vi "CS POLARIS BME DG Client.panel.vi"(8 "error in (no error)":errorcluster, 11 "object ref":refnum<vi>) -> (0 "error out":errorcluster)   [LabVIEW 2009, in "CS POLARIS BME DG Client.lvlib"]
doc: "This is the constructor of a class.\n\nLicense Agreement for this software:\n\nCopyright (C)\nGesellschaft für Schwerionenforschung, GSI\nPlanckstr. 1\n64291 Darmstadt\nGermany\n\nContact: D.Beck@gsi.de \n\nThis program is free software; you can redistribute it and/or modify it under the terms of the \nGNU General Public License as published by the Free Software Foundation; either version 2 of \nthe license, or (at your option) any later version.\n\nThis program is distributed in the hope that it will be useful, but WITHOUT ANY WARRANTY; \nwithout even the implied warranty of MERCHANTABILITY or FITNESS FOR A PARTICULAR PURPOSE. See the GNU General License for more details (http://www.gnu.org).\n\nGesellschaft für Schwerionenforschung, GSI\nPlanckstr. 1, 64291 Darmstadt, Germany\nFor all questions and ideas contact: M.Richter@gsi.de, H.Brand@gsi.de or D.Beck@gsi.de.\nLast update: 16-JUN-2004"
uses:
  CS POLARIS BME DG Client.lvlib
  CSCore/CSSystem/CoreDefs/CoreDefs.call_type.ctl
  CSCore/BaseProcess/BaseProcess.descriptor string definition.ctl
  CSCore/CSSystem/CoreDefs/CoreDefs.rawDataType.ctl
  CSCore/CSSystem/CoreLib/CoreLib.string 2 byte array.vi
  CSCore/CSSystem/CoreLib/CoreLib.byte array 2 string.vi
  CSCore/CSSystem/CoreLib/CoreLib.byte array 2 double.vi
  CSCore/CSSystem/CoreLib/CoreLib.int 2 byte array.vi
  DG Classes/BME_DG_System/ControlLevel.ctl
  CSCore/CSSystem/CSSystemLib/CSSystemLib.lvlib
  CSCore/CSSystem/CoreLib/CoreLib.lvlib
  DG Classes/BME_DG_System/BME_DG_System.lvclass
  <vilib>/gmath/NI_Gmath.lvlib
  lib.lib/UtilityLib/UtilityLib.lvlib
  CSCore/BaseProcess/BaseProcess.lvlib
panel:
  in  "deltaDelayOK":bool
  in  "call cluster in 3":T1={"Object"="", "Selector"="", "CallType"=enum."synchronous", "Async Object"="", "Async Selector"="", "Data Descriptor"="", "Data"=[], "Error #"=0, "Expire"=0}
  out "abs. Delay":dbl
  in  "call cluster in 8":T1={"Object"="", "Selector"="", "CallType"=enum."synchronous", "Async Object"="", "Async Selector"="", "Data Descriptor"="", "Data"=[], "Error #"=0, "Expire"=0}
  in  "Old Delay Formula":string
  in  "call cluster in 7":T1={"Object"="", "Selector"="", "CallType"=enum."synchronous", "Async Object"="", "Async Selector"="", "Data Descriptor"="", "Data"=[], "Error #"=0, "Expire"=0}
  in  "call cluster in 6":T1={"Object"="", "Selector"="", "CallType"=enum."synchronous", "Async Object"="", "Async Selector"="", "Data Descriptor"="", "Data"=[], "Error #"=0, "Expire"=0}
  in  "call cluster in 5":T1={"Object"="", "Selector"="", "CallType"=enum."synchronous", "Async Object"="", "Async Selector"="", "Data Descriptor"="", "Data"=[], "Error #"=0, "Expire"=0}
  in  "call cluster in 4":T1={"Object"="", "Selector"="", "CallType"=enum."synchronous", "Async Object"="", "Async Selector"="", "Data Descriptor"="", "Data"=[], "Error #"=0, "Expire"=0}
  out "Control?":bool
  in  "Tabs":enum32{"Simple", "Expert", "State"}(tab)
  out "cur. delay":dbl format="%#.9g"
  out "Ref. Chnl":string
  out "new delay":dbl format="%#.9g"
  in  "Continiously":bool
  out "Current Formula(µs)":string
  in  "ms":i32
  in  "µs":i32 min=-1000 max=1000
  in  "ns":i32 min=-1000 max=1000
  in  "Set Delay":bool
  in  "sec":i32
  in  "ps":i32 min=-1000 max=1000
  out "next common shot(s)":dbl caption="update in (s)"
  out "Out. Modulo":i32
  in  "New Modulo":i32
  in  "SetOutputMod":bool caption="Set"
  out "lockinfo":string caption="cntrl locked by"
  in  "Select ref. Chnl":u16(ring)
  out "cmd error":errorcluster
  in  "call cluster in 2":T1={"Object"="", "Selector"="", "CallType"=enum."synchronous", "Async Object"="", "Async Selector"="", "Data Descriptor"="", "Data"=[], "Error #"=0, "Expire"=0}
  in  "call cluster in":T1={"Object"="", "Selector"="", "CallType"=enum."synchronous", "Async Object"="", "Async Selector"="", "Data Descriptor"="", "Data"=[], "Error #"=0, "Expire"=0}
  out "State":i32
  out "Next Shot in (s)":dbl format="%#.1f"
  out "Rep. Rate (s)":dbl
  out "Active?":bool
  out "Channel":string
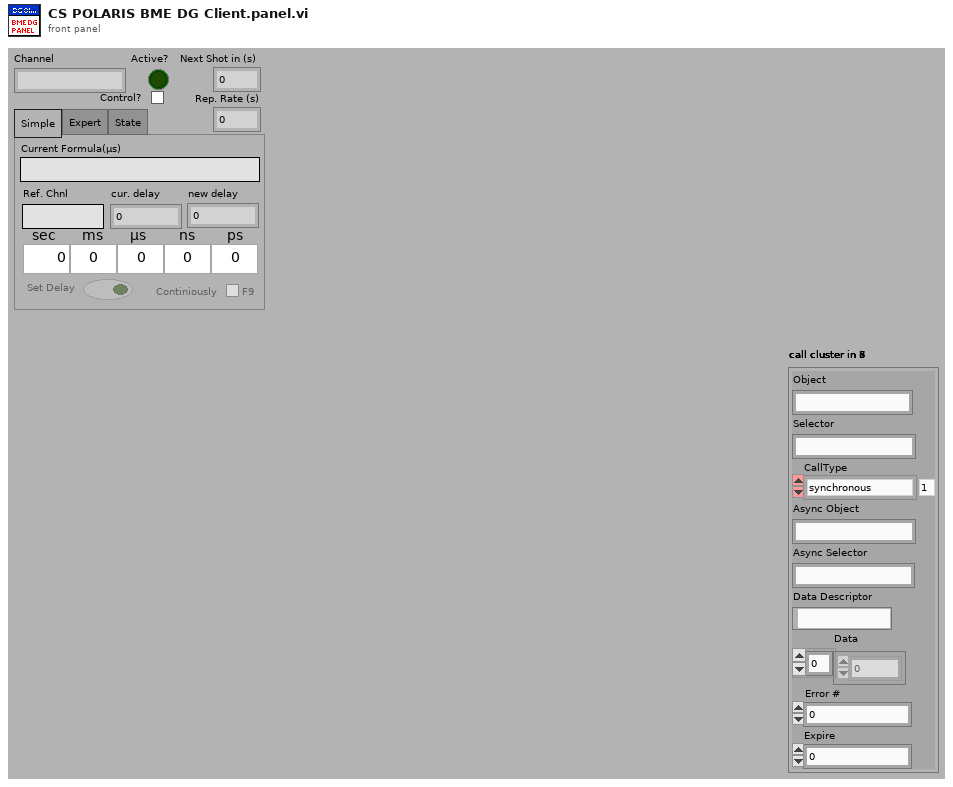
[diagram p1: front panel]
types:
  T1 = typedef "CoreDefs.call_type.ctl" = cluster{"Object":string, "Selector":string, "CallType":enum16{"simple", "synchronous", "asynchronous"}, "Async Object":string, "Async Selector":string, "Data Descriptor":T2, "Data":T3, "Error #":i32, "Expire":u32}
  T2 = typedef "BaseProcess.lvlib/BaseProcess.descriptor string definition.ctl" = string
  T3 = typedef "CoreDefs.rawDataType.ctl" = i8[]
  T4 = enum8{"Enabled", "Disabled", "Disabled and Grayed Out"}
  T5 = typedef "CS POLARIS BME DG Client.lvlib/CS POLARIS BME DG Client.i attribute.ctl" = cluster{"Delay Formula Ref":refnum<vi>, "Active Ref":refnum<vi>, "OutputModulo Ref":refnum<vi>, "Rep Rate Ref":refnum<vi>, "Next Shot Ref":refnum<vi>, "Error Ref":refnum<vi>, "Switch Ref":refnum<vi>, "New Delay Formula Ref":refnum<vi>, "New OutputModulo Ref ":refnum<vi>, "Channel":string, "CS DG Obj":string, "Stop Ref":refnum<vi>, "Max delay change":dbl, "Enabled fields":u8, "LockInfo Ref":refnum<vi>, "Next Common Shot Ref":refnum<vi>, "cur. abs del Ref":refnum<vi>, "new abs del Ref 2":refnum<vi>}
  T6 = typedef "POLARIS BME DG.lvlib/BME_DG_System.lvclass/ControlLevel.ctl" = enum16{"Simple", "Expert", "Unknown"}
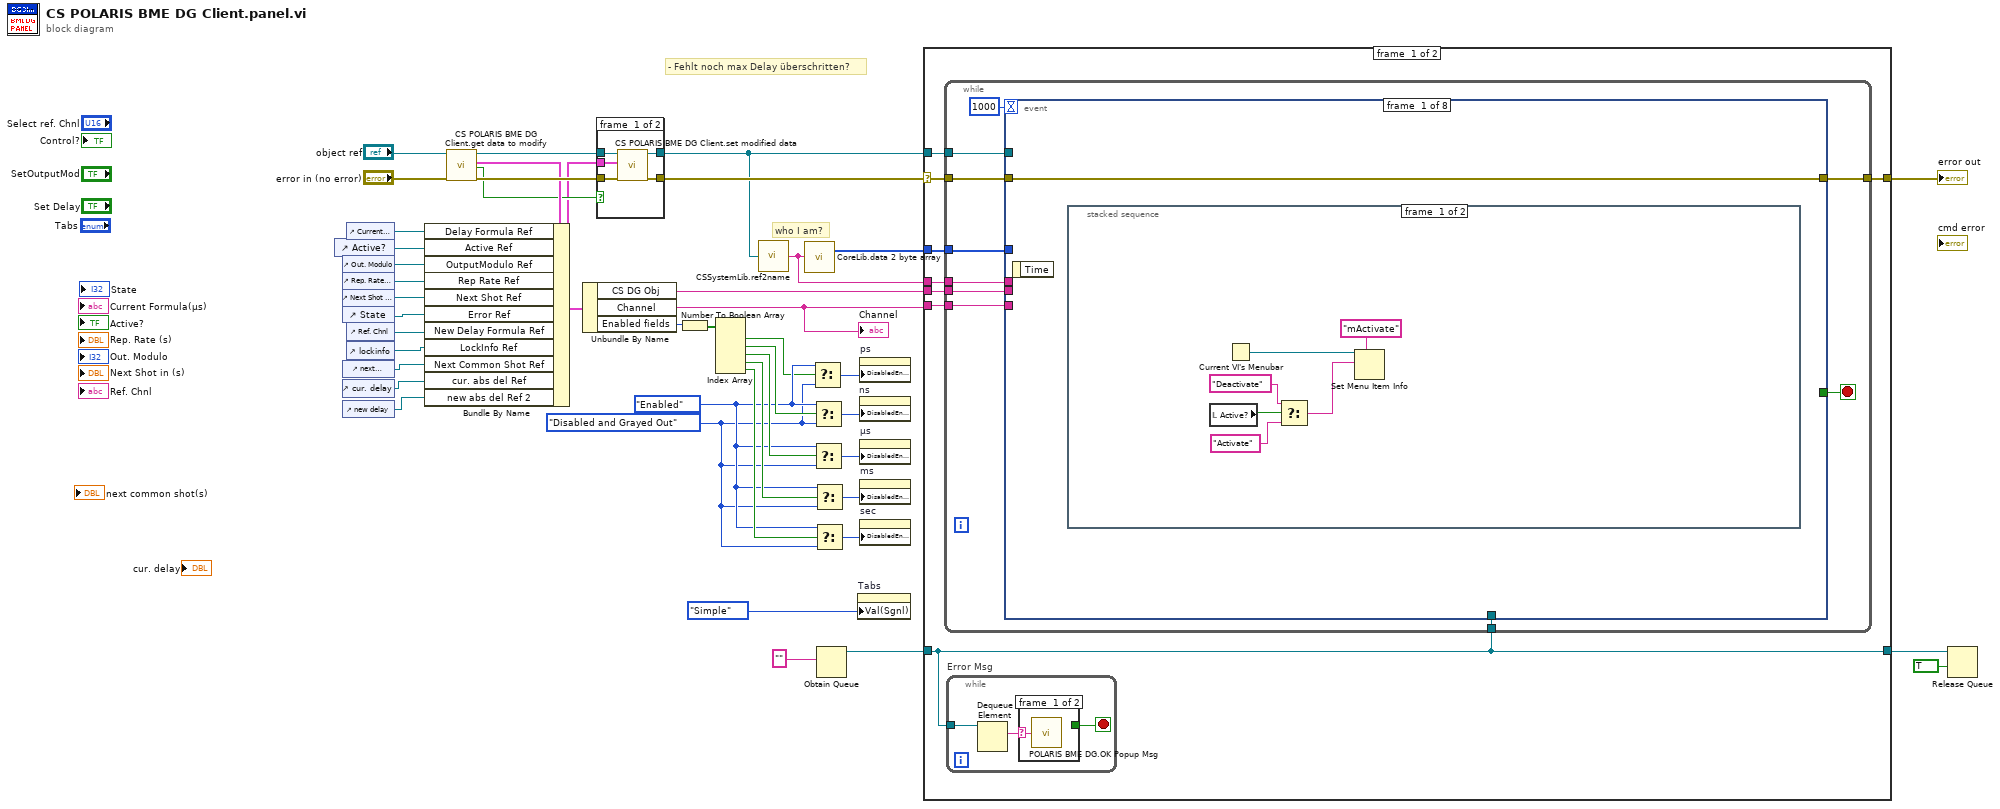
[diagram p0: block diagram]
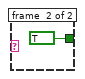
[diagram p3: hidden frame]
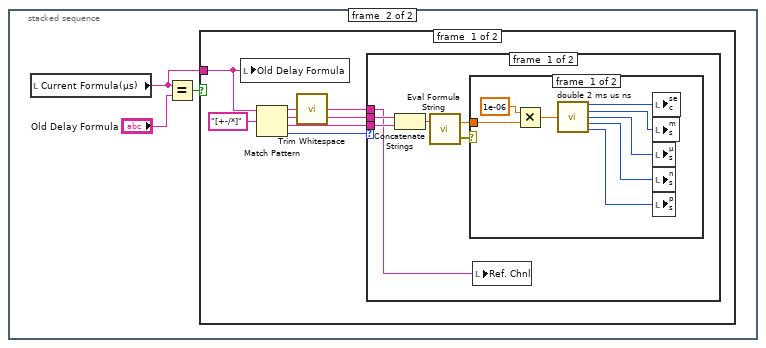
[diagram p4: hidden frame]
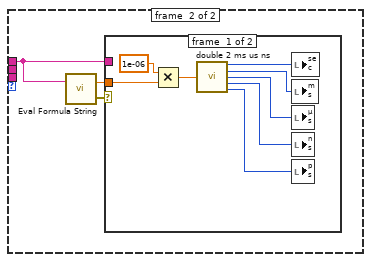
[diagram p6: hidden frame]
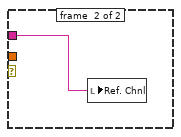
[diagram p7: hidden frame]
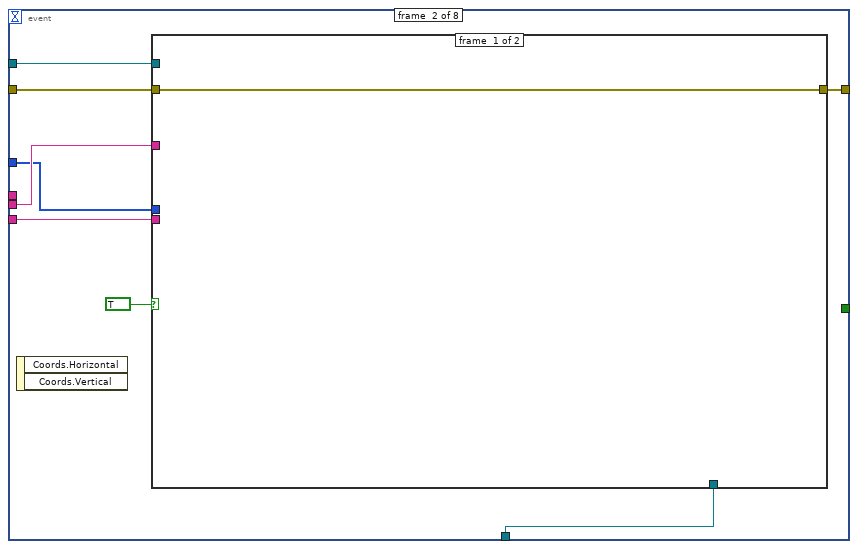
[diagram p9: hidden frame]
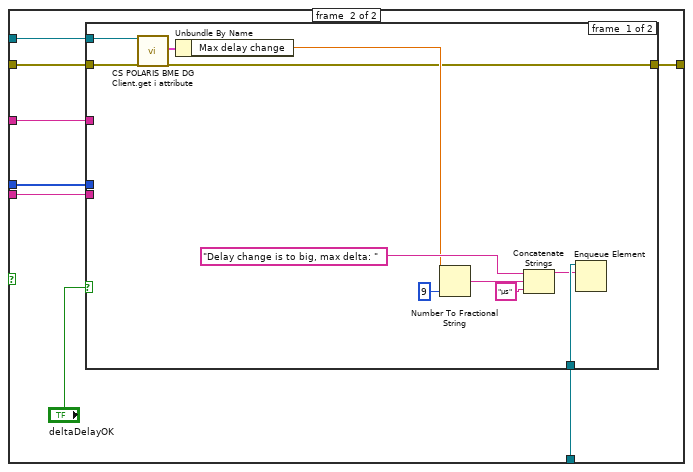
[diagram p10: hidden frame]
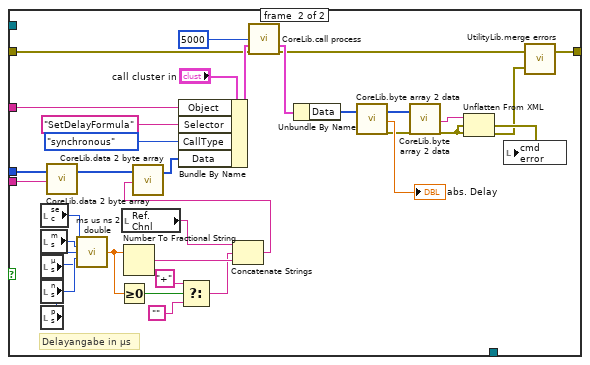
[diagram p11: hidden frame]
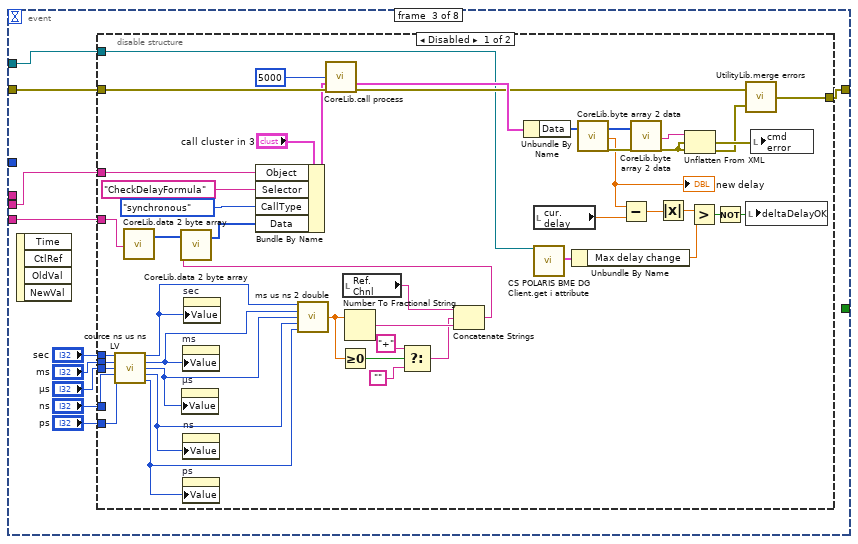
[diagram p12: hidden frame]
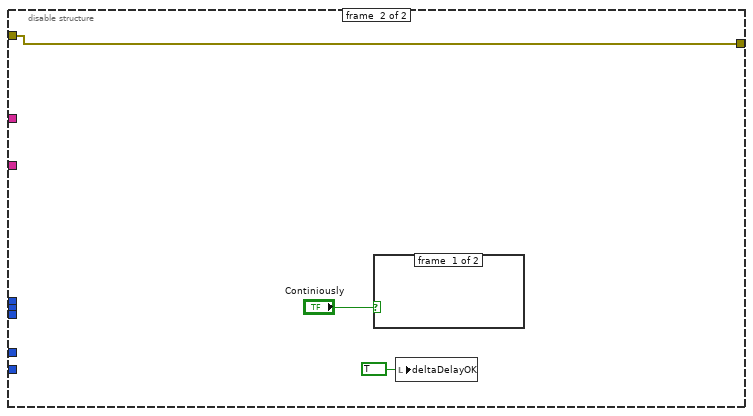
[diagram p13: hidden frame]
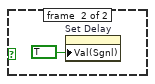
[diagram p14: hidden frame]
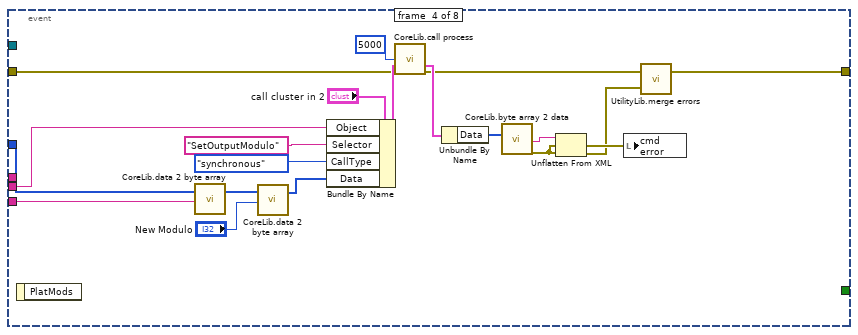
[diagram p15: hidden frame]
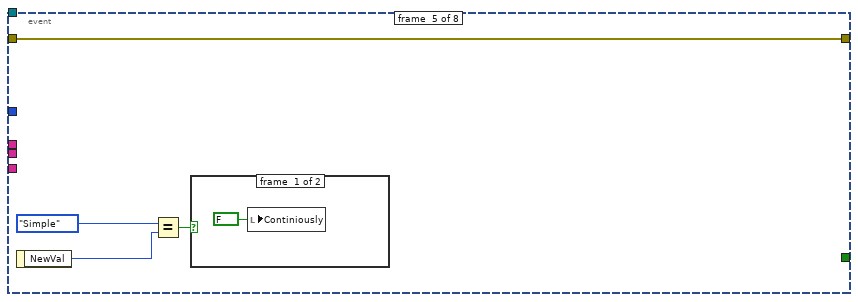
[diagram p16: hidden frame]
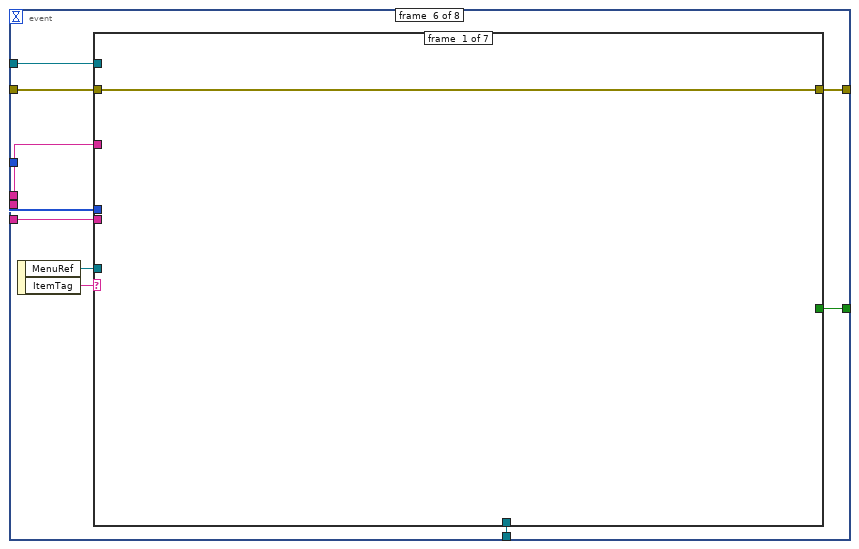
[diagram p18: hidden frame]
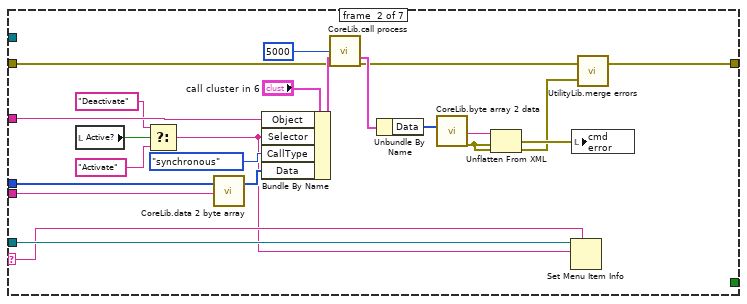
[diagram p19: hidden frame]
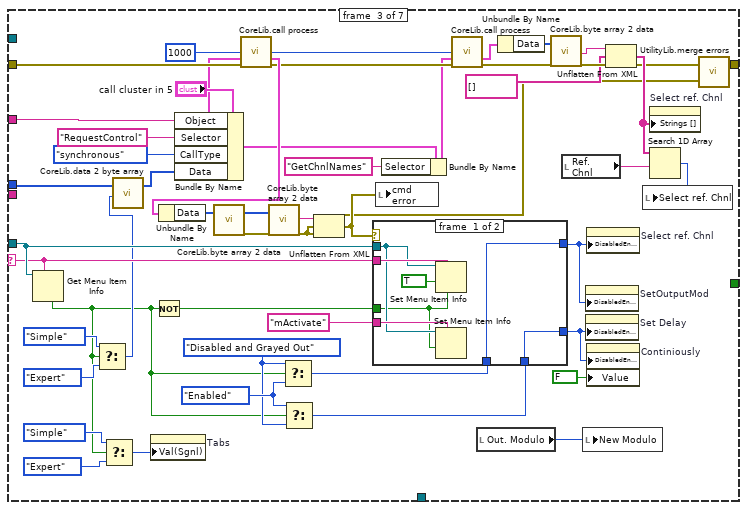
[diagram p20: hidden frame]
diagram:
  w6 = T4."Disabled and Grayed Out" ("Disabled")
  w7 = T4."Enabled" ("Disabled")
  # "who I am?"
  # "- Fehlt noch max Delay überschritten?"
  n1 = control-ref of="Active?"() -> (w33:refnum<vi>)
  n2 = control-ref of="Out. Modulo"() -> (w37:refnum<vi>)
  n3 = control-ref of="Rep. Rate (s)"() -> (w36:refnum<vi>)
  n4 = control-ref of="Next Shot in (s)"() -> (w35:refnum<vi>)
  n5 = control-ref of="State"() -> (w27:refnum<vi>)
  n6 = control-ref of="next common shot(s)"() -> (w3:refnum<vi>)
  n7 = control-ref of="cur. delay"() -> (w2:refnum<vi>)
  n8 = control-ref of="new delay"() -> (w1:refnum<vi>)
  n9 = control-ref of="Current Formula(µs)"() -> (w38:refnum<vi>)
  n10 = control-ref of="Ref. Chnl"() -> (w34:refnum<vi>)
  n11 = control-ref of="lockinfo"() -> (w18:refnum<vi>)
  n12 = call "CS POLARIS BME DG Client.get data to modify.vi"("i ref in"="object ref", "error in (no error)"="error in (no error)") -> ("i ref out"=w40:refnum<vi>, "i attribute"=w42:T5, "timed out"=w41:bool, "error out"=w43:errorcluster)  [unwired: 14 in]
  n13 = Bundle By Name(cluster=w42, "Delay Formula Ref"=w38, "Active Ref"=w33, "OutputModulo Ref"=w37, "Rep Rate Ref"=w36, "Next Shot Ref"=w35, "Error Ref"=w27, "New Delay Formula Ref"=w34, "LockInfo Ref"=w18, "Next Common Shot Ref"=w3, "cur. abs del Ref"=w2, "new abs del Ref 2"=w1) -> (w30:T5)
  n14 = Unbundle By Name(w30) -> ("CS DG Obj"=w29:string, "Channel"=w28:string, "Enabled fields"=w26:u8)
  "Channel" <- w28
  n15 = case shown="False" w41 {
    tunnel: w40 -> [w49 w51]
    tunnel: w30 -> [w48 _]
    tunnel: w43 -> [w47 w50]
    tunnel: [w46 w51] -> w22
    tunnel: [w45 w50] -> w31
    frame #0 {
      n16 = call "CS POLARIS BME DG Client.set modified data.vi"("i ref in"=w49, "i attribute"=w48, "error in (no error)"=w47) -> ("i ref out"=w46:refnum<vi>, "error out"=w45:errorcluster)  [unwired: 15 in]
    }
    frame #1 {
    }
  }
  n17 = Number To Boolean Array(number=w26) -> (Boolean array=w25:bool[])
  n18 = Index Array(array=w25) -> (element #1=w5:bool, element #2=w9:bool, element #3=w10:bool, element #4=w11:bool, element #5=w12:bool)  [unwired: 5 in]
  n19 = call "CSSystemLib.ref2name.vi"("obj refnum"=w22) -> ("name"=w19:string)
  n20 = call-poly "CoreLib.data 2 byte array.vi"("string"=w19) -> ("byteArray out"=w21:T3)  [unwired: 18 in]
  n21 = Select(t=w7, s=w5, f=w6) -> (s? t:f=w8:T4)
  n22 = Select(t=w7, s=w9, f=w6) -> (s? t:f=w23:T4)
  n23 = Select(t=w7, s=w10, f=w6) -> (s? t:f=w24:T4)
  n24 = Select(t=w7, s=w11, f=w6) -> (s? t:f=w13:T4)
  n25 = Select(t=w7, s=w12, f=w6) -> (s? t:f=w4:T4)
  n26 = Obtain Queue(element data type="") -> (queue out=w16:refnum<queue>)  [unwired: 4 in, 2 out]
  n27 = property on="Tabs" class="TabCtl (strict)"("Val(Sgnl)"=enum32{"Simple", "Expert"}."Simple" ("Tabs")) -> ()  [unwired: 2 in, 2 out]
  n28 = property on="ps" class="DigNum (strict)"("DisabledEnum"=w8) -> ()  [unwired: 2 in, 2 out]
  n29 = property on="ns" class="DigNum (strict)"("DisabledEnum"=w23) -> ()  [unwired: 2 in, 2 out]
  n30 = property on="µs" class="DigNum (strict)"("DisabledEnum"=w24) -> ()  [unwired: 2 in, 2 out]
  n31 = property on="ms" class="DigNum (strict)"("DisabledEnum"=w13) -> ()  [unwired: 2 in, 2 out]
  n32 = property on="sec" class="DigNum (strict)"("DisabledEnum"=w4) -> ()  [unwired: 2 in, 2 out]
  n33 = case shown="No Error" w31 {
    selector: w31 -> [w59 w512]
    tunnel: [w58 w512] -> w44
    tunnel: w22 -> [w57 _]
    tunnel: w29 -> [w56 _]
    tunnel: w28 -> [w55 _]
    tunnel: w21 -> [w54 _]
    tunnel: w19 -> [w53 _]
    tunnel: w16 -> [w52 w511]
    tunnel: [w52 w511] -> w15
    frame #0 {
      n34 = while {
        tunnel: w59 -> [w73]
        tunnel: [w72] -> w58
        tunnel: w57 -> [w71]
        tunnel: w56 -> [w70]
        tunnel: w55 -> [w69]
        tunnel: w54 -> [w68]
        tunnel: w53 -> [w66]
        tunnel: w52 -> [w65]
        stop <- w74 stop-if-true
        n35 = event shown="[1] \"Set Delay\": Mouse Down" {
          selector: _ -> [_ _ _ _ _ _ _ _]
          dyn-events: _ -> [_ _ _ _ _ _ _ _]
          timeout: 1000 -> [_ _ _ _ _ _ _ _]
          tunnel: [_ _ _ _ _ w269 _ _] -> w74
          tunnel: w73 -> [w75 w125 w185 w258 w265 w276 w495 w510]
          tunnel: [w75 w124 w184 w242 w265 w275 w495 w510] -> w72
          tunnel: w71 -> [_ w119 w181 _ _ w268 _ _]
          tunnel: w70 -> [_ w123 w182 w257 _ w274 _ _]
          tunnel: w69 -> [_ w122 w183 w253 _ w273 _ _]
          tunnel: w68 -> [_ w121 _ w246 _ w272 _ _]
          tunnel: w66 -> [_ _ _ _ _ _ w492 _]
          tunnel: w65 -> [_ w120 _ _ _ w267 _ _]
          event #0 {
            n36 = event-data() -> ()  [unwired: 1 in, 1 out]
            n37 = stacked-sequence {
              frame #0 {
                n38 = local read "Active?"() -> (w80:bool)
                n39 = Current VI's Menubar() -> (w81:refnum<k9>)
                n40 = Select(t="Deactivate", s=w80, f="Activate") -> (s? t:f=w77:string)
                n41 = Set Menu Item Info(7:"mActivate" ("item tag"), 10:w77, 11:w81) -> ()  [unwired: 4 in, 2 out]
              }
              frame #1 {
                n42 = local read "Current Formula(µs)"() -> (w82:string)
                n43 = Equal?(x=w82, y="Old Delay Formula") -> (x = y?=w83:bool)
                n44 = case shown="False" w83 {
                  tunnel: w82 -> [w91 _]
                  frame #0 {
                    n45 = local write "Old Delay Formula"(w91) -> ()
                    n46 = Match Pattern(string=w91, regular expression="[+-/*]") -> (before substring=w89:string, match substring=w87:string, after substring=w86:string, offset past match=w88:i32)  [unwired: 1 in]
                    n47 = call <vilib>:"Trim Whitespace.vi"("string"=w89) -> ("trimmed string"=w85:string)  [unwired: 1 in]
                    n48 = case shown="0, Default" w88 {
                      tunnel: w87 -> [w97 _]
                      tunnel: w86 -> [w96 _]
                      tunnel: w85 -> [w92 w106]
                      frame #0 {
                        n49 = Concatenate Strings(w97, w96) -> (w95:string)
                        n50 = call <vilib>:"Eval Formula String.vi"("formula"=w95) -> ("error out"=w93:errorcluster, "y value"=w94:dbl)  [unwired: 1 in]
                        n51 = case shown="No Error" w93 {
                          tunnel: w94 -> [w105 _]
                          frame #0 {
                            n52 = Multiply(x=1e-06, y=w105) -> (x*y=w104:dbl)
                            n53 = call "double 2 ms us ns.vi"("sec"=w104) -> ("sec"=w98:i32, "ms"=w102:i32, "µs"=w101:i32, "ns"=w100:i32, "ps"=w99:i32)  [unwired: 10 in]
                            n54 = local write "sec"(w98) -> ()
                            n55 = local write "ms"(w102) -> ()
                            n56 = local write "µs"(w101) -> ()
                            n57 = local write "ns"(w100) -> ()
                            n58 = local write "ps"(w99) -> ()
                          }
                          frame #1 {
                          }
                        }
                        n59 = local write "Ref. Chnl"(w92) -> ()
                      }
                      frame #1 {
                        n60 = call <vilib>:"Eval Formula String.vi"("formula"=w106) -> ("error out"=w108:errorcluster, "y value"=w107:dbl)  [unwired: 1 in]
                        n61 = case shown="No Error" w108 {
                          tunnel: w107 -> [w116 _]
                          tunnel: w106 -> [_ w117]
                          frame #0 {
                            n62 = Multiply(x=1e-06, y=w116) -> (x*y=w109:dbl)
                            n63 = call "double 2 ms us ns.vi"("sec"=w109) -> ("sec"=w111:i32, "ms"=w114:i32, "µs"=w113:i32, "ns"=w112:i32, "ps"=w110:i32)  [unwired: 10 in]
                            n64 = local write "sec"(w111) -> ()
                            n65 = local write "ms"(w114) -> ()
                            n66 = local write "µs"(w113) -> ()
                            n67 = local write "ns"(w112) -> ()
                            n68 = local write "ps"(w110) -> ()
                          }
                          frame #1 {
                            n69 = local write "Ref. Chnl"(w117) -> ()
                          }
                        }
                      }
                    }
                  }
                  frame #1 {
                  }
                }
              }
            }
          }
          event #1 {
            n70 = event-data() -> ()  [unwired: 1 in, 2 out]
            n71 = case shown="True" TRUE {
              tunnel: w125 -> [w126 w134]
              tunnel: [w126 w130] -> w124
              tunnel: w123 -> [_ w133]
              tunnel: w122 -> [_ w132]
              tunnel: w121 -> [_ w131]
              tunnel: w120 -> [_ w128]
              tunnel: w119 -> [_ w127]
              frame #0 {
              }
              frame #1 {
                n72 = case shown="True" "deltaDelayOK" {
                  tunnel: w134 -> [w140 w177]
                  tunnel: w133 -> [_ w176]
                  tunnel: w132 -> [_ w168]
                  tunnel: w131 -> [_ w164]
                  tunnel: [w139 w153] -> w130
                  tunnel: w128 -> [w145 _]
                  tunnel: w127 -> [w141 _]
                  frame #0 {
                    n73 = call "CS POLARIS BME DG Client.get i attribute.vi"("i ref in"=w141, "error in (no error)"=w140) -> ("i attribute"=w143:T5, "error out"=w139:errorcluster)  [unwired: 15 in, 1 out]
                    n74 = Unbundle By Name(w143) -> ("Max delay change"=w142:dbl)
                    n75 = Number To Fractional String(number=w142, precision (6)=i16 9) -> (F-format string=w136:string)  [unwired: 2 in]
                    n76 = Concatenate Strings("Delay change is to big, max delta: " ("element"), w136, "µs" ("string")) -> (w138:string)
                    n77 = Enqueue Element(queue=w145, element=w138) -> ()  [unwired: 2 in, 3 out]
                  }
                  frame #1 {
                    # "Delayangabe in µs"
                    n78 = local read "sec"() -> (w150:i32)
                    n79 = local read "ms"() -> (w163:i32)
                    n80 = local read "µs"() -> (w162:i32)
                    n81 = local read "ns"() -> (w161:i32)
                    n82 = local read "ps"() -> (w151:i32)
                    n83 = call-poly "CoreLib.data 2 byte array.vi"("byteArray"=w164, "string"=w168) -> ("byteArray out"=w173:T3)  [unwired: 17 in]
                    n84 = call "ms us ns 2 double.vi"("sec"=w150, "ms"=w163, "µs"=w162, "ns"=w161, "ps"=w151) -> ("µs"=w160:dbl)  [unwired: 10 in]
                    n85 = Greater Or Equal To 0?(x=w160) -> (x >= 0?=w159:bool)
                    n86 = local read "Ref. Chnl"() -> (w167:string)
                    n87 = Number To Fractional String(number=w160) -> (F-format string=w165:string)  [unwired: 3 in]
                    n88 = Select(t="+", s=w159, f="") -> (s? t:f=w156:string)
                    n89 = Concatenate Strings(w167, w156, w165) -> (w166:string)
                    n90 = call-poly "CoreLib.data 2 byte array.vi"("byteArray"=w173, "string"=w166) -> ("byteArray out"=w172:T3)  [unwired: 17 in]
                    n91 = Bundle By Name(cluster="call cluster in", "Object"=w176, "Selector"="SetDelayFormula", "CallType"=enum16{"simple", "synchronous", "asynchronous"}."synchronous", "Data"=w172) -> (w180:T1)
                    n92 = call "CoreLib.call process.vi"("timeout (ms)"=5000, "call cluster in"=w180, "error in (no error)"=w177) -> ("call cluster out"=w171:T1, "error out"=w154:errorcluster)  [unwired: 11 in]
                    n93 = Unbundle By Name(w171) -> ("Data"=w149:T3)
                    n94 = call-poly "CoreLib.byte array 2 data.vi"("byteArray"=w149) -> ("byteArray out"=w148:T3, "d64"=→"abs. Delay":dbl, "error out"=w146:errorcluster)  [unwired: 16 in]
                    n95 = call-poly "CoreLib.byte array 2 data.vi"("byteArray"=w148, "error in (no error)"=w146) -> ("string"=w170:string, "error out"=w169:errorcluster)  [unwired: 15 in, 1 out]
                    n96 = Unflatten From XML(xml string=w170, type=w169, error in (no error)=w169) -> (value=w155:errorcluster, error out=w152:errorcluster)
                    n97 = local write "cmd error"(w155) -> ()
                    n98 = call "UtilityLib.merge errors.vi"("error2 (no error)"=w152, "error1 (no error)"=w154) -> ("error out"=w153:errorcluster)
                  }
                }
              }
            }
          }
          event #2 {
            n99 = event-data() -> ()  [unwired: 1 in, 4 out]
            n100 = disable-structure shown="Disabled" {
              disable-tunnel: "sec" -> [w237 _]
              disable-tunnel: "ms" -> [w236 _]
              disable-tunnel: "µs" -> [w235 _]
              disable-tunnel: "ns" -> [w234 _]
              disable-tunnel: "ps" -> [w233 _]
              disable-tunnel: w185 -> [w232 w240]
              disable-tunnel: [w202 w240] -> w184
              disable-tunnel: w183 -> [w201 _]
              disable-tunnel: w182 -> [w200 _]
              disable-tunnel: w181 -> [w195 _]
              frame #0 {
                n101 = call "cource ns us ns LV.vi"("sec in"=w237, "ms in"=w236, "µs in"=w235, "ns in"=w234, "ps in"=w233) -> ("sec out"=w231:i32, "ms out"=w230:i32, "µs out"=w229:i32, "ns out"=w204:i32, "ps out"=w203:i32)  [unwired: 6 in]
                n102 = call-poly "CoreLib.data 2 byte array.vi"("string"=w201) -> ("byteArray out"=w223:T3)  [unwired: 18 in]
                n103 = property on="µs" class="DigNum (strict)"("Value"=w229) -> ()  [unwired: 2 in, 2 out]
                n104 = property on="ms" class="DigNum (strict)"("Value"=w230) -> ()  [unwired: 2 in, 2 out]
                n105 = property on="ns" class="DigNum (strict)"("Value"=w204) -> ()  [unwired: 2 in, 2 out]
                n106 = property on="ps" class="DigNum (strict)"("Value"=w203) -> ()  [unwired: 2 in, 2 out]
                n107 = property on="sec" class="DigNum (strict)"("Value"=w231) -> ()  [unwired: 2 in, 2 out]
                n108 = call "ms us ns 2 double.vi"("sec"=w231, "ms"=w230, "µs"=w229, "ns"=w204, "ps"=w203) -> ("µs"=w215:dbl)  [unwired: 10 in]
                n109 = Greater Or Equal To 0?(x=w215) -> (x >= 0?=w214:bool)
                n110 = local read "Ref. Chnl"() -> (w218:string)
                n111 = Number To Fractional String(number=w215) -> (F-format string=w216:string)  [unwired: 3 in]
                n112 = Select(t="+", s=w214, f="") -> (s? t:f=w211:string)
                n113 = Concatenate Strings(w218, w211, w216) -> (w217:string)
                n114 = call-poly "CoreLib.data 2 byte array.vi"("byteArray"=w223, "string"=w217) -> ("byteArray out"=w222:T3)  [unwired: 17 in]
                n115 = Bundle By Name(cluster="call cluster in 3", "Object"=w200, "Selector"="CheckDelayFormula", "CallType"=enum16{"simple", "synchronous", "asynchronous"}."synchronous", "Data"=w222) -> (w228:T1)
                n116 = call "CoreLib.call process.vi"("timeout (ms)"=5000, "call cluster in"=w228, "error in (no error)"=w232) -> ("call cluster out"=w221:T1, "error out"=w209:errorcluster)  [unwired: 11 in]
                n117 = Unbundle By Name(w221) -> ("Data"=w207:T3)
                n118 = local read "cur. delay"() -> (w199:dbl)
                n119 = call "CS POLARIS BME DG Client.get i attribute.vi"("i ref in"=w195) -> ("i attribute"=w194:T5)  [unwired: 16 in, 2 out]
                n120 = Unbundle By Name(w194) -> ("Max delay change"=w193:dbl)
                n121 = call-poly "CoreLib.byte array 2 data.vi"("byteArray"=w207) -> ("byteArray out"=w206:T3, "d64"=w198:dbl, "error out"=w205:errorcluster)  [unwired: 16 in]
                "new delay" <- w198
                n122 = Subtract(x=w198, y=w199) -> (x-y=w197:dbl)
                n123 = call-poly "CoreLib.byte array 2 data.vi"("byteArray"=w206, "error in (no error)"=w205) -> ("string"=w220:string, "error out"=w219:errorcluster)  [unwired: 15 in, 1 out]
                n124 = Absolute Value(x=w197) -> (abs(x)=w196:dbl)
                n125 = Unflatten From XML(xml string=w220, type=w219, error in (no error)=w219) -> (value=w210:errorcluster, error out=w208:errorcluster)
                n126 = Greater?(x=w196, y=w193) -> (0:w192:bool)
                n127 = Not(x=w192) -> (.not. x?=w191:bool)
                n128 = call "UtilityLib.merge errors.vi"("error2 (no error)"=w208, "error1 (no error)"=w209) -> ("error out"=w202:errorcluster)
                n129 = local write "deltaDelayOK"(w191) -> ()
                n130 = local write "cmd error"(w210) -> ()
              }
              frame #1 {
                n131 = case shown="True" "Continiously" {
                  frame #0 {
                  }
                  frame #1 {
                    n132 = property on="Set Delay" class="Bool (strict)"("Val(Sgnl)"=TRUE ("Value (Signaling)")) -> ()  [unwired: 2 in, 2 out]
                  }
                }
                n133 = local write "deltaDelayOK"(TRUE ("deltaDelayOK")) -> ()
              }
            }
          }
          event #3 {
            n134 = event-data() -> ()  [unwired: 1 in, 1 out]
            n135 = call-poly "CoreLib.data 2 byte array.vi"("byteArray"=w246, "string"=w253) -> ("byteArray out"=w254:T3)  [unwired: 17 in]
            n136 = call-poly "CoreLib.data 2 byte array.vi"("byteArray"=w254, "i32"="New Modulo") -> ("byteArray out"=w252:T3)  [unwired: 17 in]
            n137 = Bundle By Name(cluster="call cluster in 2", "Object"=w257, "Selector"="SetOutputModulo", "CallType"=enum16{"simple", "synchronous", "asynchronous"}."synchronous", "Data"=w252) -> (w261:T1)
            n138 = call "CoreLib.call process.vi"("timeout (ms)"=5000, "call cluster in"=w261, "error in (no error)"=w258) -> ("call cluster out"=w251:T1, "error out"=w243:errorcluster)  [unwired: 11 in]
            n139 = Unbundle By Name(w251) -> ("Data"=w250:T3)
            n140 = call-poly "CoreLib.byte array 2 data.vi"("byteArray"=w250) -> ("string"=w249:string, "error out"=w248:errorcluster)  [unwired: 16 in, 1 out]
            n141 = Unflatten From XML(xml string=w249, type=w248, error in (no error)=w248) -> (value=w245:errorcluster, error out=w244:errorcluster)
            n142 = local write "cmd error"(w245) -> ()
            n143 = call "UtilityLib.merge errors.vi"("error2 (no error)"=w244, "error1 (no error)"=w243) -> ("error out"=w242:errorcluster)
          }
          event #4 {
            n144 = event-data() -> ("NewVal"=w263:enum32{"Simple", "Expert", "State"})  [unwired: 1 in]
            n145 = Equal?(x=enum32{"Simple", "Expert"}."Simple" ("NewVal"), y=w263) -> (x = y?=w262:bool)
            n146 = case shown="False" w262 {
              frame #0 {
                n147 = local write "Continiously"(FALSE ("Continiously")) -> ()
              }
              frame #1 {
              }
            }
          }
          event #5 {
            n148 = event-data() -> ("MenuRef"=w270:refnum<k9>, "ItemTag"=w271:string)  [unwired: 1 in]
            n149 = case shown="\"mReleaseCntrl\"" w271 {
              selector: w271 -> [_ w284 w324 w373 _ _ _]
              tunnel: w276 -> [w277 w297 w339 w378 w422 w449 w472]
              tunnel: [w277 w278 w302 w366 w413 w448 w459] -> w275
              tunnel: w274 -> [_ w296 w338 w377 w421 _ w471]
              tunnel: w273 -> [_ w294 _ _ _ _ _]
              tunnel: w272 -> [_ w286 w340 w380 w409 _ w473]
              tunnel: w270 -> [_ w285 w325 w372 w406 _ w461]
              tunnel: [_ _ _ _ _ TRUE _] -> w269
              tunnel: w268 -> [_ _ _ _ _ w450 _]
              tunnel: w267 -> [_ _ _ w360 w404 w447 w453]
              frame #0 {
              }
              frame #1 {
                n150 = local read "Active?"() -> (w282:bool)
                n151 = Select(t="Deactivate" ("Selector"), s=w282, f="Activate" ("Selector")) -> (s? t:f=w283:string)
                n152 = call-poly "CoreLib.data 2 byte array.vi"("byteArray"=w286, "string"=w294) -> ("byteArray out"=w293:T3)  [unwired: 17 in]
                n153 = Bundle By Name(cluster="call cluster in 6", "Object"=w296, "Selector"=w283, "CallType"=enum16{"simple", "synchronous", "asynchronous"}."synchronous", "Data"=w293) -> (w300:T1)
                n154 = call "CoreLib.call process.vi"("timeout (ms)"=5000, "call cluster in"=w300, "error in (no error)"=w297) -> ("call cluster out"=w292:T1, "error out"=w279:errorcluster)  [unwired: 11 in]
                n155 = Unbundle By Name(w292) -> ("Data"=w291:T3)
                n156 = call-poly "CoreLib.byte array 2 data.vi"("byteArray"=w291) -> ("string"=w290:string, "error out"=w289:errorcluster)  [unwired: 16 in, 1 out]
                n157 = Unflatten From XML(xml string=w290, type=w289, error in (no error)=w289) -> (value=w281:errorcluster, error out=w280:errorcluster)
                n158 = Set Menu Item Info(7:w284, 10:w283, 11:w285) -> ()  [unwired: 4 in, 2 out]
                n159 = local write "cmd error"(w281) -> ()
                n160 = call "UtilityLib.merge errors.vi"("error2 (no error)"=w280, "error1 (no error)"=w279) -> ("error out"=w278:errorcluster)
              }
              frame #2 {
                w316 = T4."Enabled" ("Disabled")
                w315 = T4."Disabled and Grayed Out" ("Disabled")
                w336 = 1000 ("timeout (ms)")
                n161 = Get Menu Item Info(7:w324, 11:w325) -> (4:w308:bool)  [unwired: 1 in, 6 out]
                n162 = Select(t=ControlLevel."Simple" ("Control level"), s=w308, f=ControlLevel."Expert" ("Control level")) -> (s? t:f=w311:T6)
                n163 = Select(t=enum32{"Simple", "Expert"}."Simple" ("Value (Signaling)"), s=w308, f=enum32{"Simple", "Expert"}."Expert" ("Value (Signaling)")) -> (s? t:f=w307:enum32{"Simple", "Expert"})
                n164 = call-poly "CoreLib.data 2 byte array.vi"("byteArray"=w340, "i32"=w311) -> ("byteArray out"=w348:T3)  [unwired: 17 in]
                n165 = property on="Tabs" class="TabCtl (strict)"("Val(Sgnl)"=w307) -> ()  [unwired: 2 in, 2 out]
                n166 = Not(x=w308) -> (.not. x?=w321:bool)
                n167 = Bundle By Name(cluster="call cluster in 5", "Object"=w338, "Selector"="RequestControl", "CallType"=enum16{"simple", "synchronous", "asynchronous"}."synchronous", "Data"=w348) -> (w335:T1)
                n168 = call "CoreLib.call process.vi"("timeout (ms)"=w336, "call cluster in"=w335, "error in (no error)"=w339) -> ("call cluster out"=w347:T1, "error out"=w337:errorcluster)  [unwired: 11 in]
                n169 = Unbundle By Name(w347) -> ("Data"=w344:T3)
                n170 = call-poly "CoreLib.byte array 2 data.vi"("byteArray"=w344) -> ("byteArray out"=w343:T3, "error out"=w342:errorcluster)  [unwired: 16 in, 1 out]
                n171 = call-poly "CoreLib.byte array 2 data.vi"("byteArray"=w343, "error in (no error)"=w342) -> ("string"=w346:string, "error out"=w345:errorcluster)  [unwired: 15 in, 1 out]
                n172 = Select(t=w315, s=w308, f=w316) -> (s? t:f=w319:T4)
                n173 = Select(t=w316, s=w308, f=w315) -> (s? t:f=w317:T4)
                n174 = Unflatten From XML(xml string=w346, type=w345, error in (no error)=w345) -> (value=w305:errorcluster, error out=w304:errorcluster)
                n175 = case shown="Error" w305 {
                  tunnel: [w357 w359] -> w318
                  tunnel: w319 -> [w356 _]
                  tunnel: w317 -> [w357 _]
                  tunnel: [w356 w359] -> w306
                  tunnel: w325 -> [w352 _]
                  tunnel: w324 -> [w354 _]
                  tunnel: "mActivate" ("item tag") -> [w353 _]
                  tunnel: w321 -> [w351 _]
                  frame #0 {
                    n176 = Set Menu Item Info(6:w351, 7:w354, 9:TRUE ("enabled"), 11:w352) -> ()  [unwired: 3 in, 2 out]
                    n177 = Set Menu Item Info(7:w353, 9:w351, 11:w352) -> ()  [unwired: 4 in, 2 out]
                  }
                  frame #1 {
                    w359 = T4."Disabled and Grayed Out" ("Disabled")
                    n178 = local write "Control?"(FALSE ("Control?")) -> ()
                  }
                }
                n179 = local write "cmd error"(w305) -> ()
                n180 = Bundle By Name(cluster=w335, "Selector"="GetChnlNames") -> (w333:T1)
                n181 = call "CoreLib.call process.vi"("timeout (ms)"=w336, "call cluster in"=w333, "error in (no error)"=w337) -> ("call cluster out"=w332:T1, "error out"=w327:errorcluster)  [unwired: 11 in]
                n182 = local read "Out. Modulo"() -> (w320:i32)
                n183 = Unbundle By Name(w332) -> ("Data"=w331:T3)
                n184 = call-poly "CoreLib.byte array 2 data.vi"("byteArray"=w331, "error in (no error)"=w327) -> ("string"=w328:string, "error out"=w330:errorcluster)  [unwired: 15 in, 1 out]
                n185 = local read "Ref. Chnl"() -> (w313:string)
                n186 = local write "New Modulo"(w320) -> ()
                n187 = property on="SetOutputMod" class="Bool (strict)"("DisabledEnum"=w306) -> ()  [unwired: 2 in, 2 out]
                n188 = property on="Set Delay" class="Bool (strict)"("DisabledEnum"=w318) -> ()  [unwired: 2 in, 2 out]
                n189 = property on="Select ref. Chnl" class="Ring (strict)"("DisabledEnum"=w306) -> ()  [unwired: 2 in, 2 out]
                n190 = property on="Continiously" class="Bool (strict)"("DisabledEnum"=w318, "Value"=FALSE ("Continiously")) -> ()  [unwired: 2 in, 2 out]
                n191 = Unflatten From XML(xml string=w328, type=string[] [], error in (no error)=w330) -> (value=w314:string[], error out=w303:errorcluster)
                n192 = property on="Select ref. Chnl" class="Ring (strict)"("Strings []"=w314) -> ()  [unwired: 2 in, 2 out]
                n193 = Search 1D Array(1D array=w314, element=w313) -> (index of element=w312:i32)  [unwired: 1 in]
                n194 = local write "Select ref. Chnl"(w312) -> ()
                n195 = call "UtilityLib.merge errors.vi"("error2 (no error)"=w304, "error1 (no error)"=w303) -> ("error out"=w302:errorcluster)
              }
              frame #3 {
                w381 = T4."Disabled and Grayed Out" ("Disabled")
                n196 = Set Menu Item Info(7:"mRequestExpertCtrl" ("item name"), 9:TRUE ("enabled"), 11:w372) -> ()  [unwired: 4 in, 2 out]
                n197 = Set Menu Item Info(7:w373, 9:FALSE ("checked"), 11:w372) -> ()  [unwired: 4 in, 2 out]
                n198 = call-poly "CoreLib.data 2 byte array.vi"("byteArray"=w380, "i32"=ControlLevel."Simple" ("Control level")) -> ("byteArray out"=w390:T3)  [unwired: 17 in]
                n199 = local write "Tabs"(enum32{"Simple", "Expert"}."Simple" ("Tabs")) -> ()
                n200 = Bundle By Name(cluster="call cluster in 4", "Object"=w377, "Selector"="RequestControl", "CallType"=enum16{"simple", "synchronous", "asynchronous"}."synchronous", "Data"=w390) -> (w394:T1)
                n201 = call "CoreLib.call process.vi"("timeout (ms)"=1000, "call cluster in"=w394, "error in (no error)"=w378) -> ("call cluster out"=w389:T1, "error out"=w367:errorcluster)  [unwired: 11 in]
                n202 = Unbundle By Name(w389) -> ("Data"=w385:T3)
                n203 = call-poly "CoreLib.byte array 2 data.vi"("byteArray"=w385) -> ("byteArray out"=w384:T3, "string"=w363:string, "error out"=w383:errorcluster)  [unwired: 16 in]
                "lockinfo" <- w363
                n204 = call-poly "CoreLib.byte array 2 data.vi"("byteArray"=w384, "error in (no error)"=w383) -> ("string"=w388:string, "error out"=w387:errorcluster)  [unwired: 15 in, 1 out]
                n205 = Unflatten From XML(xml string=w388, type=w387, error in (no error)=w387) -> (value=w365:errorcluster, error out=w368:errorcluster)
                n206 = case shown="Error" w365 {
                  tunnel: [w396 T4."Disabled and Grayed Out" ("Disabled")] -> w382
                  tunnel: T4."Enabled" ("Disabled") -> [w396 _]
                  tunnel: [TRUE _] -> w370
                  tunnel: w363 -> [_ w401]
                  tunnel: "Control is locked by:  " ("item name") -> [_ w400]
                  tunnel: "; try force control  " ("item name") -> [_ w399]
                  tunnel: w360 -> [_ w398]
                  frame #0 {
                  }
                  frame #1 {
                    n207 = Concatenate Strings(w400, w401, w399) -> (w397:string)
                    n208 = local write "Control?"(FALSE ("Control?")) -> ()
                    n209 = Enqueue Element(queue=w398, element=w397) -> ()  [unwired: 2 in, 3 out]
                  }
                }
                n210 = local write "Control?"(w370) -> ()
                n211 = property on="Continiously" class="Bool (strict)"("DisabledEnum"=w382, "Value"=FALSE ("Continiously")) -> ()  [unwired: 2 in, 2 out]
                n212 = property on="Set Delay" class="Bool (strict)"("DisabledEnum"=w382) -> ()  [unwired: 2 in, 2 out]
                n213 = property on="Select ref. Chnl" class="Ring (strict)"("DisabledEnum"=w381) -> ()  [unwired: 2 in, 2 out]
                n214 = property on="SetOutputMod" class="Bool (strict)"("DisabledEnum"=w381) -> ()  [unwired: 2 in, 2 out]
                n215 = call "UtilityLib.merge errors.vi"("error2 (no error)"=w368, "error1 (no error)"=w367) -> ("error out"=w366:errorcluster)
                n216 = local write "cmd error"(w365) -> ()
              }
              frame #4 {
                w424 = T4."Disabled and Grayed Out" ("Disabled")
                n217 = Set Menu Item Info(7:"mRequestSimpleCntrl" ("item tag"), 9:FALSE ("checked"), 11:w406) -> ()  [unwired: 4 in, 2 out]
                n218 = Set Menu Item Info(7:"mRequestExpertCtrl" ("item name"), 9:TRUE ("enabled"), 11:w406) -> ()  [unwired: 4 in, 2 out]
                n219 = local write "Tabs"(enum32{"Simple", "Expert"}."Simple" ("Tabs")) -> ()
                n220 = Bundle By Name(cluster="call cluster in 8", "Object"=w421, "Selector"="ForceControl", "CallType"=enum16{"simple", "synchronous", "asynchronous"}."synchronous", "Data"=w409) -> (w435:T1)
                n221 = call "CoreLib.call process.vi"("timeout (ms)"=1000, "call cluster in"=w435, "error in (no error)"=w422) -> ("call cluster out"=w431:T1, "error out"=w414:errorcluster)  [unwired: 11 in]
                n222 = Unbundle By Name(w431) -> ("Data"=w428:T3)
                n223 = call-poly "CoreLib.byte array 2 data.vi"("byteArray"=w428) -> ("byteArray out"=w427:T3, "string"=w408:string, "error out"=w426:errorcluster)  [unwired: 16 in]
                n224 = call-poly "CoreLib.byte array 2 data.vi"("byteArray"=w427, "error in (no error)"=w426) -> ("string"=w430:string, "error out"=w429:errorcluster)  [unwired: 15 in, 1 out]
                n225 = local write "lockinfo"(w408) -> ()
                n226 = Unflatten From XML(xml string=w430, type=w429, error in (no error)=w429) -> (value=w412:errorcluster, error out=w415:errorcluster)
                n227 = case shown="No Error" w412 {
                  tunnel: [w438 T4."Disabled and Grayed Out" ("Disabled")] -> w425
                  tunnel: T4."Enabled" ("Disabled") -> [w438 _]
                  tunnel: [TRUE _] -> w417
                  tunnel: w408 -> [_ w443]
                  tunnel: "Force Control error, DG are still locked by:  " ("item name") -> [_ w442]
                  tunnel: w404 -> [w436 w441]
                  tunnel: [w436 w439] -> _
                  frame #0 {
                  }
                  frame #1 {
                    n228 = Concatenate Strings(w442, w443) -> (w440:string)
                    n229 = local write "Control?"(FALSE ("Control?")) -> ()
                    n230 = Enqueue Element(queue=w441, element=w440) -> (queue out=w439:refnum<queue>)  [unwired: 2 in, 2 out]
                  }
                }
                n231 = local write "Control?"(w417) -> ()
                n232 = property on="Continiously" class="Bool (strict)"("DisabledEnum"=w425, "Value"=FALSE ("Continiously")) -> ()  [unwired: 2 in, 2 out]
                n233 = property on="Set Delay" class="Bool (strict)"("DisabledEnum"=w425) -> ()  [unwired: 2 in, 2 out]
                n234 = property on="Select ref. Chnl" class="Ring (strict)"("DisabledEnum"=w424) -> ()  [unwired: 2 in, 2 out]
                n235 = property on="SetOutputMod" class="Bool (strict)"("DisabledEnum"=w424) -> ()  [unwired: 2 in, 2 out]
                n236 = call "UtilityLib.merge errors.vi"("error2 (no error)"=w415, "error1 (no error)"=w414) -> ("error out"=w413:errorcluster)
                n237 = local write "cmd error"(w412) -> ()
              }
              frame #5 {
                n238 = call "CSSystemLib.ref2name.vi"("obj refnum"=w450) -> ("name"=w451:string)
                n239 = call "CSSystemLib._delete_nw.vi"("objectName"=w451, "error in (no error)"=w449) -> ("error out"=w448:errorcluster)  [unwired: 17 in]
                n240 = Enqueue Element(queue=w447, element="Ciao!") -> ()  [unwired: 2 in, 3 out]
              }
              frame #6 {
                w467 = FALSE ("enabled")
                w469 = T4."Disabled and Grayed Out" ("Disabled")
                n241 = Set Menu Item Info(6:w467, 7:"mRequestExpertCtrl" ("item name"), 9:w467, 11:w461) -> ()  [unwired: 3 in, 2 out]
                n242 = Set Menu Item Info(7:"mActivate" ("item tag"), 9:FALSE ("enabled"), 11:w461) -> ()  [unwired: 4 in, 2 out]
                n243 = Set Menu Item Info(7:"mRequestSimpleCntrl" ("item name"), 9:TRUE ("enabled"), 11:w461) -> ()  [unwired: 4 in, 2 out]
                n244 = Bundle By Name(cluster="call cluster in 7", "Object"=w471, "Selector"="ReleaseControl", "CallType"=enum16{"simple", "synchronous", "asynchronous"}."synchronous", "Data"=w473) -> (w484:T1)
                n245 = local write "Control?"(FALSE ("Control?")) -> ()
                n246 = call "CoreLib.call process.vi"("timeout (ms)"=1000, "call cluster in"=w484, "error in (no error)"=w472) -> ("call cluster out"=w480:T1, "error out"=w460:errorcluster)  [unwired: 11 in]
                n247 = Unbundle By Name(w480) -> ("Data"=w477:T3)
                n248 = call-poly "CoreLib.byte array 2 data.vi"("byteArray"=w477) -> ("byteArray out"=w476:T3, "string"=w454:string, "error out"=w475:errorcluster)  [unwired: 16 in]
                n249 = local write "lockinfo"(w454) -> ()
                n250 = call-poly "CoreLib.byte array 2 data.vi"("byteArray"=w476, "error in (no error)"=w475) -> ("string"=w479:string, "error out"=w478:errorcluster)  [unwired: 15 in, 1 out]
                n251 = Unflatten From XML(xml string=w479, type=w478, error in (no error)=w478) -> (value=w457:errorcluster, error out=w458:errorcluster)
                n252 = case shown="Error" w457 {
                  tunnel: [w485 T4."Disabled and Grayed Out" ("Disabled")] -> w474
                  tunnel: w469 -> [w485 _]
                  tunnel: "Release Error: System still loced by: " ("string") -> [_ w489]
                  tunnel: w454 -> [_ w488]
                  tunnel: w453 -> [_ w487]
                  frame #0 {
                  }
                  frame #1 {
                    n253 = Concatenate Strings(w489, w488) -> (w486:string)
                    n254 = local write "Control?"(FALSE ("Control?")) -> ()
                    n255 = Enqueue Element(queue=w487, element=w486) -> ()  [unwired: 2 in, 3 out]
                  }
                }
                n256 = property on="Set Delay" class="Bool (strict)"("DisabledEnum"=w474) -> ()  [unwired: 2 in, 2 out]
                n257 = property on="Select ref. Chnl" class="Ring (strict)"("DisabledEnum"=w469) -> ()  [unwired: 2 in, 2 out]
                n258 = property on="SetOutputMod" class="Bool (strict)"("DisabledEnum"=w469) -> ()  [unwired: 2 in, 2 out]
                n259 = property on="Continiously" class="Bool (strict)"("DisabledEnum"=w474, "Value"=FALSE ("Continiously")) -> ()  [unwired: 2 in, 2 out]
                n260 = local write "cmd error"(w457) -> ()
                n261 = call "UtilityLib.merge errors.vi"("error2 (no error)"=w458, "error1 (no error)"=w460) -> ("error out"=w459:errorcluster)
              }
            }
          }
          event #6 {
            n262 = event-data() -> ("NewVal"=w494:string)  [unwired: 1 in]
            n263 = Not Equal?(x=w492, y=w494) -> (x != y?=w493:bool)
            n264 = case shown="True" w493 {
              frame #0 {
              }
              frame #1 {
                w503 = FALSE ("enabled")
                w505 = T4."Disabled and Grayed Out" ("Disabled")
                n265 = Current VI's Menubar() -> (w497:refnum<k9>)
                n266 = Set Menu Item Info(6:w503, 7:"mRequestExpertCtrl" ("item name"), 9:w503, 11:w497) -> ()  [unwired: 3 in, 2 out]
                n267 = Set Menu Item Info(7:"mActivate" ("item tag"), 9:FALSE ("enabled"), 11:w497) -> ()  [unwired: 4 in, 2 out]
                n268 = Set Menu Item Info(7:"mRequestSimpleCntrl" ("item name"), 9:TRUE ("enabled"), 11:w497) -> ()  [unwired: 4 in, 2 out]
                n269 = property on="Continiously" class="Bool (strict)"("DisabledEnum"=w505, "Value"=FALSE ("Continiously")) -> ()  [unwired: 2 in, 2 out]
                n270 = property on="Set Delay" class="Bool (strict)"("DisabledEnum"=w505) -> ()  [unwired: 2 in, 2 out]
                n271 = property on="Select ref. Chnl" class="Ring (strict)"("DisabledEnum"=w505) -> ()  [unwired: 2 in, 2 out]
                n272 = property on="SetOutputMod" class="Bool (strict)"("DisabledEnum"=w505) -> ()  [unwired: 2 in, 2 out]
                n273 = local write "Control?"(FALSE ("Control?")) -> ()
              }
            }
          }
          event #7 {
            n274 = event-data() -> ("NewVal"=w508:u16)  [unwired: 1 in]
            n275 = property on="Select ref. Chnl" class="Ring (strict)"() -> ("Strings []"=w509:string[])  [unwired: 2 in, 2 out]
            n276 = Index Array(array=w509, index=w508) -> (element=w507:string)
            n277 = local write "Continiously"(FALSE ("Continiously")) -> ()
            n278 = property on="Ref. Chnl" class="Str"("Val(Sgnl)"=w507) -> ()  [unwired: 2 in, 2 out]
          }
        }
      }
      n279 = while "Error Msg" {
        tunnel: w52 -> [w62]
        stop <- w60 stop-if-true
        n280 = Dequeue Element(queue=w62) -> (element=w61:string)  [unwired: 2 in, 3 out]
        n281 = case shown="Default" w61 {
          selector: w61 -> [w63 _]
          tunnel: [_ TRUE] -> w60
          frame #0 {
            n282 = call "POLARIS BME DG.OK Popup Msg.vi"("Msg"=w63) -> ()  [unwired: 3 in]
          }
          frame #1 {
          }
        }
      }
    }
    frame #1 {
    }
  }
  "error out" <- w44
  n283 = Release Queue(queue=w15, force destroy? (F)=TRUE) -> ()  [unwired: 1 in, 3 out]
